vi "PV Main.vi"(10 "Data DVRs":T1, 11 "Config Folder":path) -> ()   [LabVIEW 2018]
uses:
  <vilib>/ORNL/CSEISMIC DDS/CSEISMIC DDS Base/Data Types/Controls/DeviceID.ctl
  Controls/DDS State.ctl
  Controls/Data Type DVRs.ctl
  <vilib>/ORNL/CSEISMIC DDS/CSEISMIC DDS Base/Data Types/IED_Status.ctl
  <vilib>/ORNL/CSEISMIC DDS/CSEISMIC DDS Base/Data Types/Controls/Timestamp.ctl
  <vilib>/ORNL/CSEISMIC DDS/CSEISMIC DDS Base/Data Types/DER_Control.ctl
  <vilib>/ORNL/CSEISMIC DDS/CSEISMIC DDS Base/Data Types/DER_SetPointP.ctl
  <vilib>/ORNL/CSEISMIC DDS/CSEISMIC DDS Base/Data Types/DER_SetPointQ.ctl
  <vilib>/ORNL/CSEISMIC DDS/CSEISMIC DDS Base/Data Types/DER_Measurement.ctl
  <vilib>/ORNL/CSEISMIC DDS/CSEISMIC DDS Base/Data Types/DER_Status.ctl
  <vilib>/ORNL/CSEISMIC DDS/CSEISMIC DDS Base/Data Types/Controls/DroopCurve.ctl
  1ea38d0c-38a7-4a3d-ae1e-65f6e0254380.vi
  8ec4fbad-6e5c-457e-b0e3-a341ac60e8a3.vi
  0ef71f9b-3bca-4440-a5c8-8282c2586051.vi
  9f7c2006-f978-4bec-9c38-bdd34ecae6aa.vi
  3fc4b4bd-7c90-499c-9ed9-e822aa1def77.vi
  ea58e506-6616-4327-a77b-3af52f62fbc1.vi
  89549c33-b0cf-467c-b5c7-b685aa9ebbb0.vi
  4802f4bd-dba4-4fda-a24e-999c1f9497bc.vi
  3edf557d-cbb6-4b9c-94ed-0284affd1f65.vi
  Global Variables/Stop (Global).vi
  Global Variables/DDS States (Global).vi
  Global Variables/Broadcast Topics (Global).vi
  Global Variables/Measurements (Global).vi
  Global Variables/Timeout Topics (Global).vi
  <vilib>/ORNL/CSEISMIC DDS/CSEISMIC DDS Base/CSEISMIC DDS.lvclass
panel:
  out "P_ref":sgl
  out "Q_ref":sgl
  out "P_meas":sgl
  out "Q_meas":sgl
  out "MicrogridID":u8
  out "Error in DDS Loop":bool
  out "DDS Loop error out":errorcluster
  out "PV DDS State":T2=enum."Shutdown"
  out "DDS loop time":u32=105
  out "DeviceID":T3
  out "Enable INV A":bool
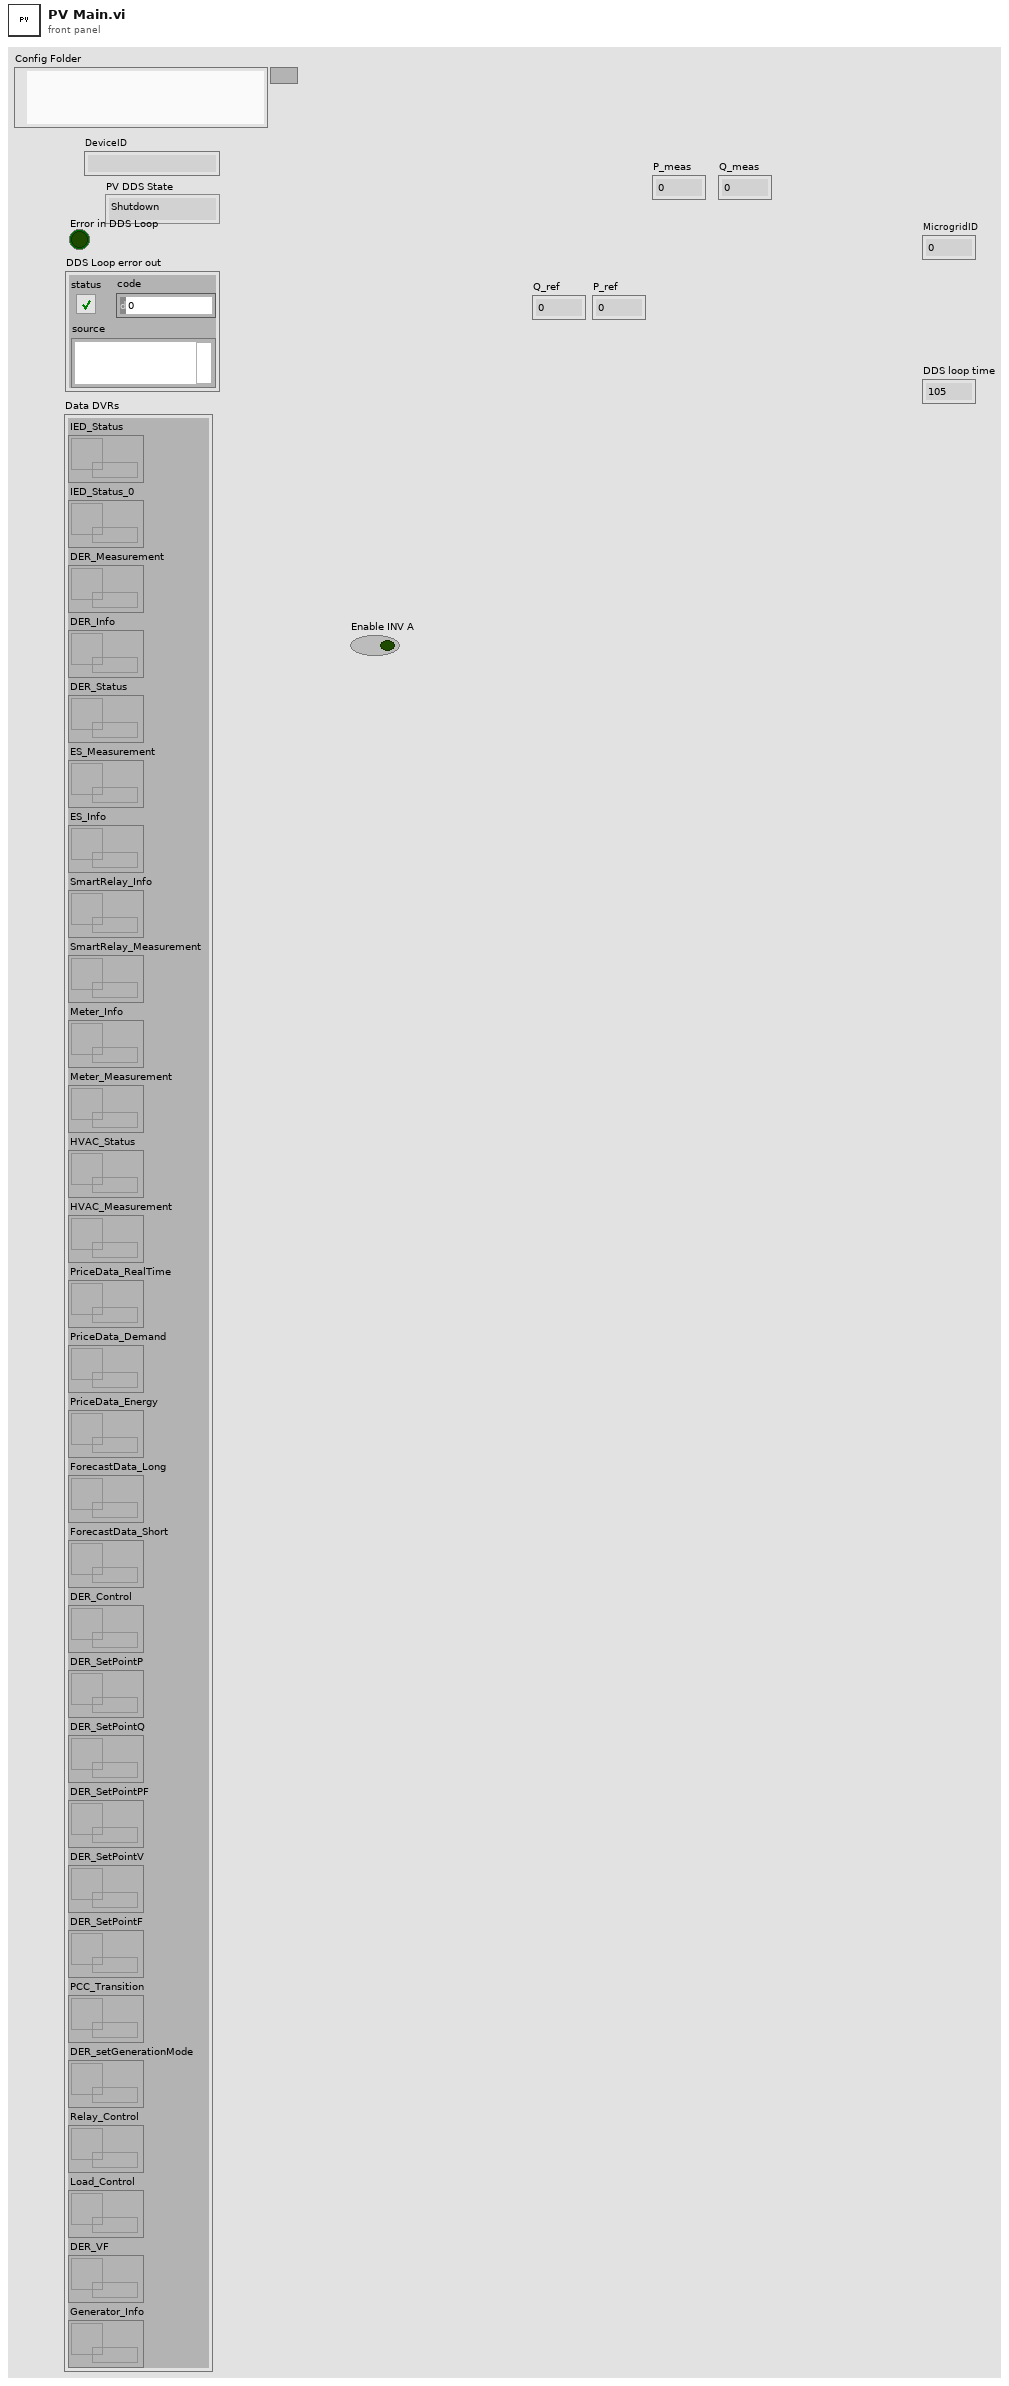
[diagram p1: front panel]
types:
  T1 = typedef "Data Type DVRs.ctl" = cluster{"IED_Status":refnum<data-value>, "IED_Status_0":refnum<data-value>, "DER_Measurement":refnum<data-value>, "DER_Info":refnum<data-value>, "DER_Status":refnum<data-value>, "ES_Measurement":refnum<data-value>, "ES_Info":refnum<data-value>, "SmartRelay_Info":refnum<data-value>, "SmartRelay_Measurement":refnum<data-value>, "Meter_Info":refnum<data-value>, "Meter_Measurement":refnum<data-value>, "HVAC_Status":refnum<data-value>, "HVAC_Measurement":refnum<data-value>, "PriceData_RealTime":refnum<data-value>, "PriceData_Demand":refnum<data-value>, "PriceData_Energy":refnum<data-value>, "ForecastData_Long":refnum<data-value>, "ForecastData_Short":refnum<data-value>, "DER_Control":refnum<data-value>, "DER_SetPointP":refnum<data-value>, "DER_SetPointQ":refnum<data-value>, "DER_SetPointPF":refnum<data-value>, "DER_SetPointV":refnum<data-value>, "DER_SetPointF":refnum<data-value>, "PCC_Transition":refnum<data-value>, "DER_setGenerationMode":refnum<data-value>, "Relay_Control":refnum<data-value>, "Load_Control":refnum<data-value>, "DER_VF":refnum<data-value>, "Generator_Info":refnum<data-value>}
  T2 = typedef "DDS State.ctl" = enum16{"Commissioning", "CheckID", "InitDDS", "ReadDDS", "WriteDDS", "CheckClose", "Close", "Shutdown"}
  T3 = typedef "CSEISMIC DDS.lvlib/CSEISMIC DDS.lvclass/DeviceID.ctl" = string
  T4 = typedef "Scaling Coefficients Cluster.ctl" = cluster{"Measurements":T5, "Setpoints":T6}
  T5 = typedef "Scaling Coefficients Measurements.ctl" = cluster{"Current":dbl, "Voltage":dbl, "Real Power":dbl, "Reactive Power":dbl, "SOC":dbl}
  T6 = typedef "Scaling Coefficients Setpoints.ctl" = cluster{"Voltage":dbl, "Frequency":dbl, "Real Power":dbl, "Reactive Power":dbl}
  T7 = typedef "CSEISMIC DDS.lvlib/CSEISMIC DDS.lvclass/DER_Info.ctl" = cluster{"DeviceID":T3, "LineConfig":u8[], "NominalVoltage(V)":dbl, "PowerRating(kVA)":dbl, "VFControl":bool, "PControl":bool, "QControl":bool, "PFControl":bool, "PVControl":bool, "Droop":bool, "DroopConfigurable":bool, "Unbalanced":bool}
  T8 = typedef "CSEISMIC DDS.lvlib/CSEISMIC DDS.lvclass/Timestamp.ctl" = cluster{"Seconds":u64, "Remainder":u64}
  T9 = typedef "CSEISMIC DDS.lvlib/CSEISMIC DDS.lvclass/IED_Status.ctl" = cluster{"DeviceID":T3, "Timestamp":T8, "MicrogridID":u8, "Active":bool, "Inactive":bool, "Error":i32, "Fault":bool, "ErrorString":string}
  T10 = typedef "CSEISMIC DDS.lvlib/CSEISMIC DDS.lvclass/DER_SetPointQ.ctl" = cluster{"DeviceID":T3, "ReactivePower (kVAR)":dbl[]}
  T11 = typedef "CSEISMIC DDS.lvlib/CSEISMIC DDS.lvclass/DER_SetPointP.ctl" = cluster{"DeviceID":T3, "RealPower (kW)":dbl[]}
  T12 = typedef "CSEISMIC DDS.lvlib/CSEISMIC DDS.lvclass/DER_Control.ctl" = cluster{"DeviceID":T3, "Activate":bool, "Deactivate":bool}
  T13 = typedef "CSEISMIC DDS.lvlib/CSEISMIC DDS.lvclass/DER_Status.ctl" = cluster{"DeviceID":T3, "VFControl":bool, "PControl":bool, "QControl":bool, "PFControl":bool, "PVControl":bool, "Droop":bool, "Unbalanced":bool, "MicrogridVF":bool, "RealDroop(kW)":T14, "ReactiveDroop(kVar)":T14}
  T14 = typedef "CSEISMIC DDS.lvlib/CSEISMIC DDS.lvclass/DroopCurve.ctl" = cluster{"XMin":dbl, "XMax":dbl, "YMin":dbl, "YMax":dbl}
  T15 = typedef "CSEISMIC DDS.lvlib/CSEISMIC DDS.lvclass/DER_Measurement.ctl" = cluster{"DeviceID":T3, "Voltage":dbl[], "Current":dbl[], "RealPower":dbl[], "ReactivePower":dbl[], "LineConfig":u8[], "Frequency":dbl}
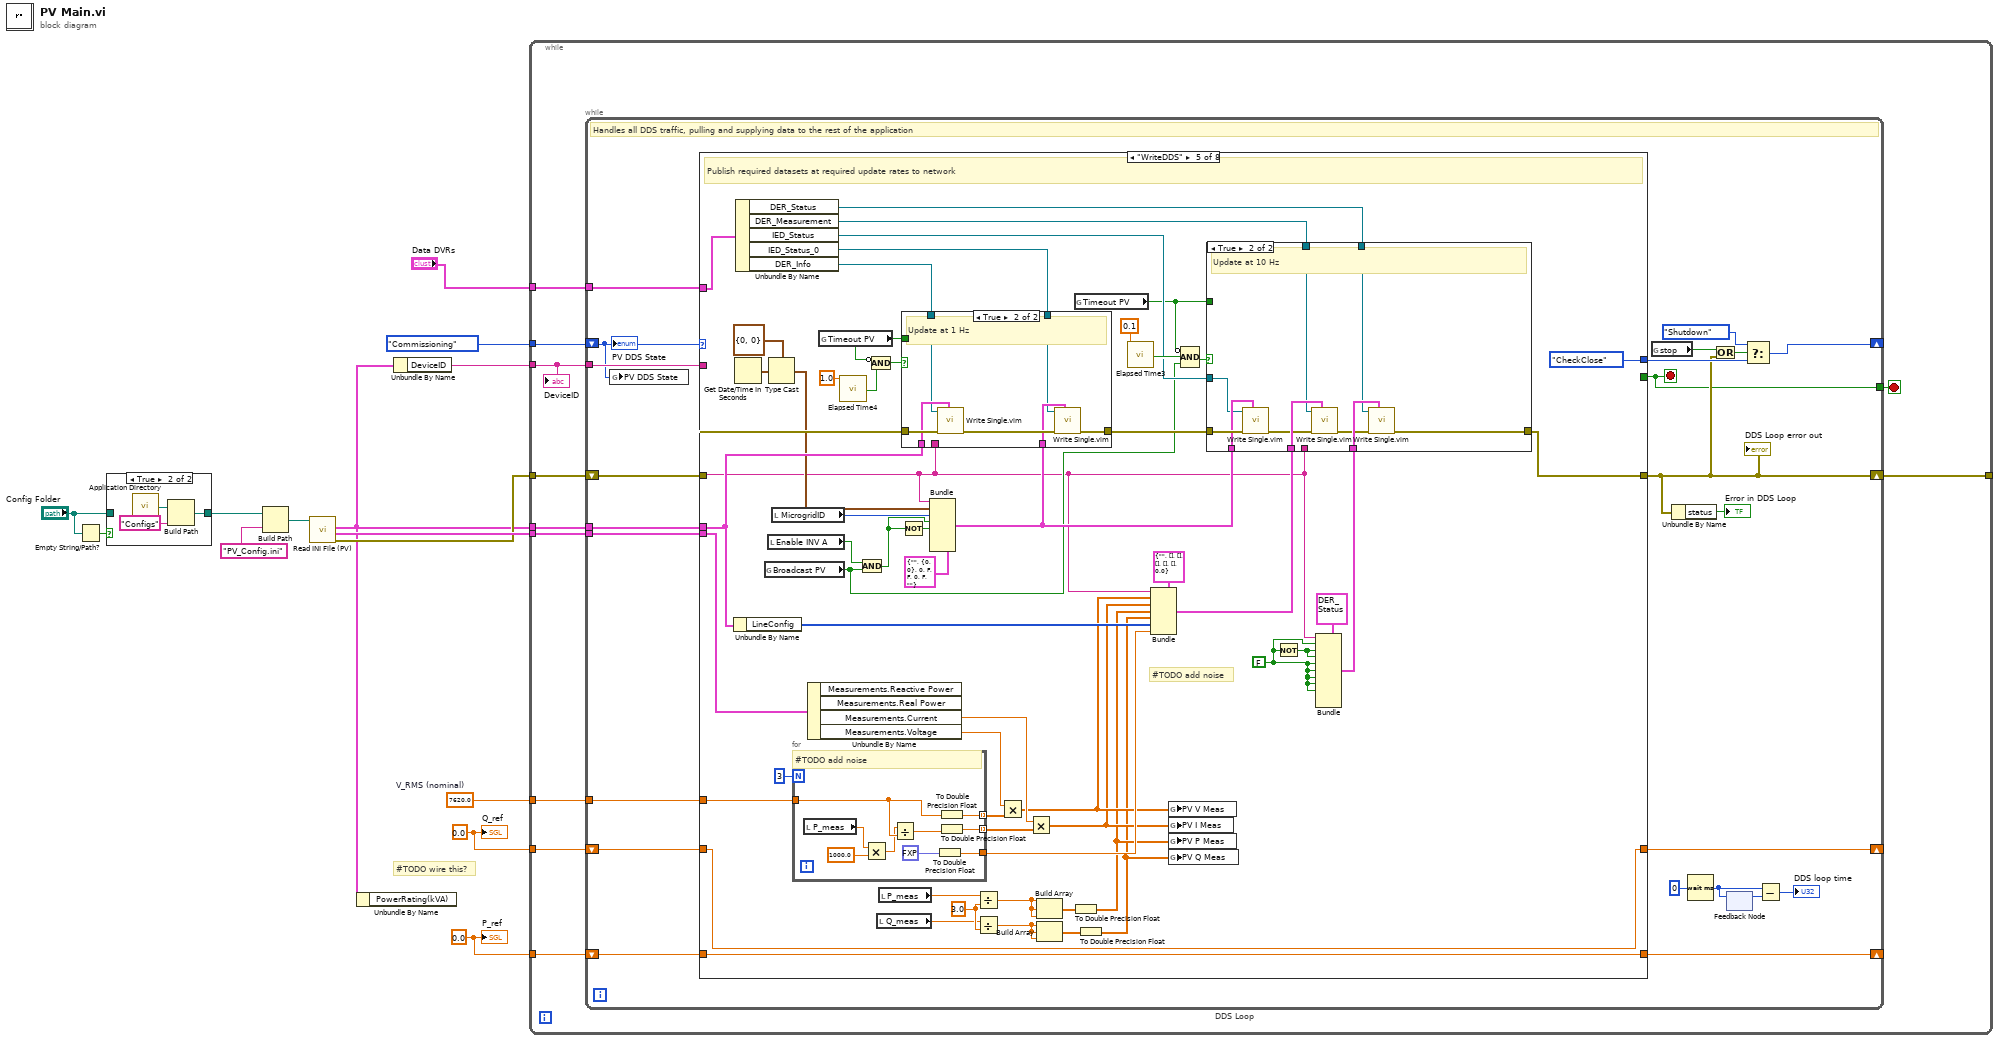
[diagram p0: block diagram]
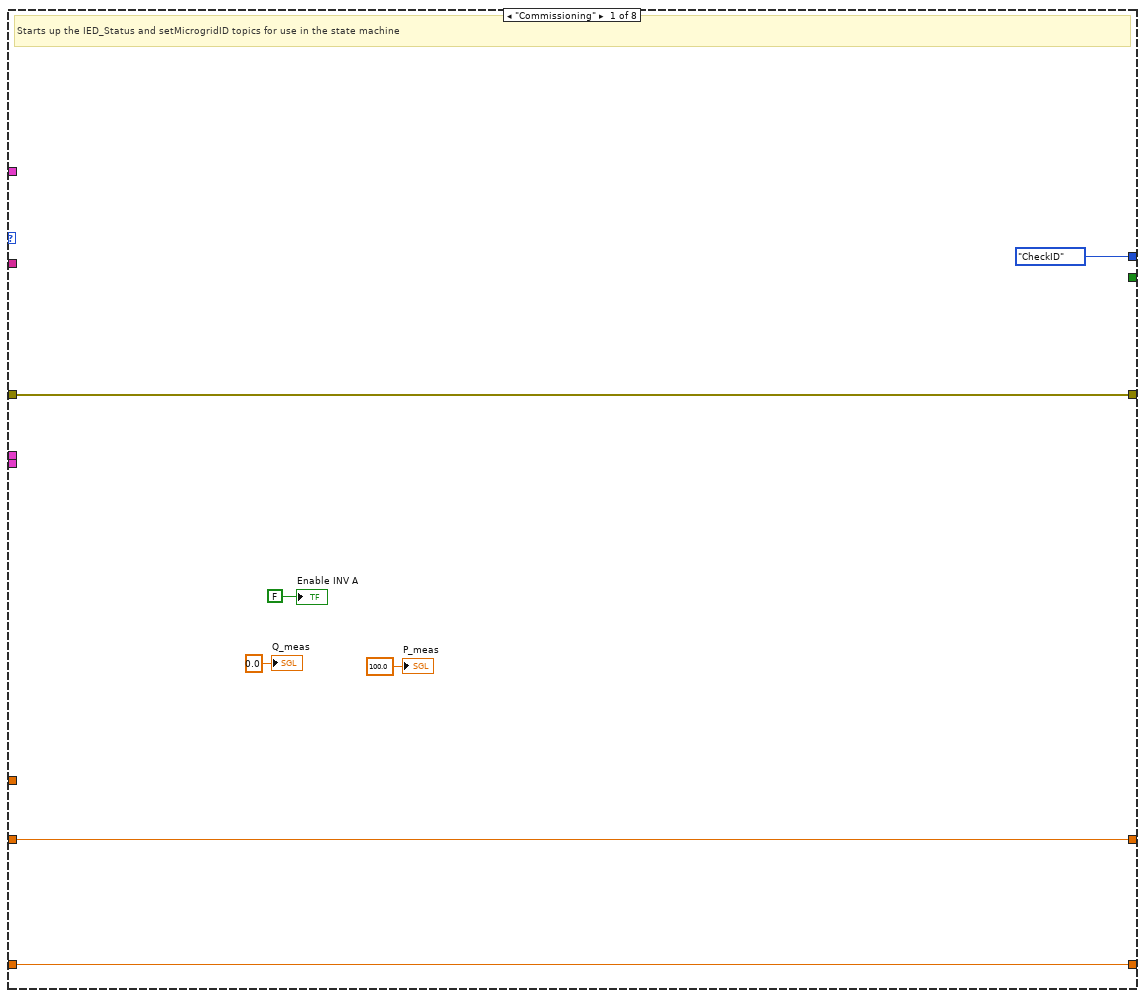
[diagram p2: hidden frame]
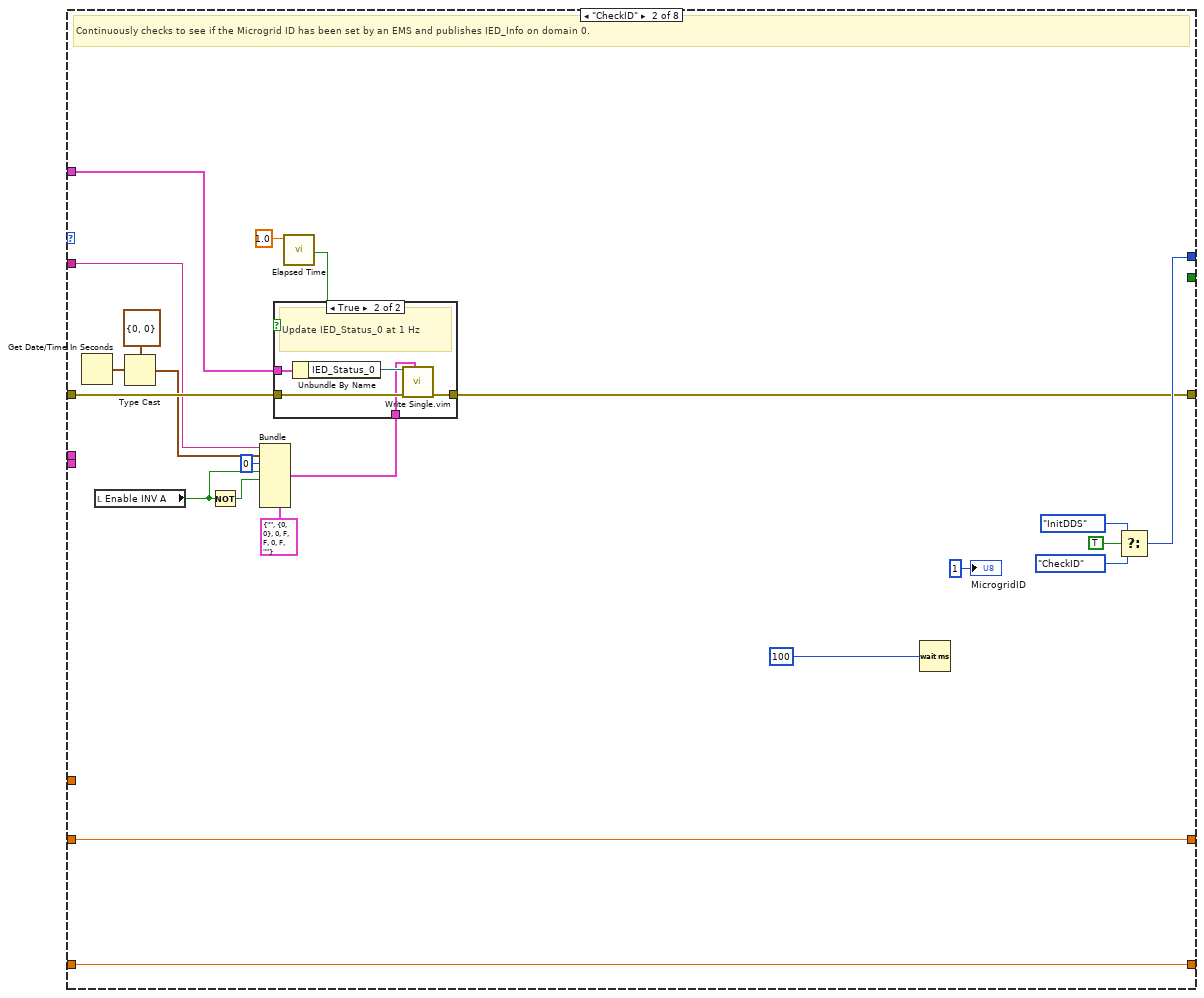
[diagram p3: hidden frame]
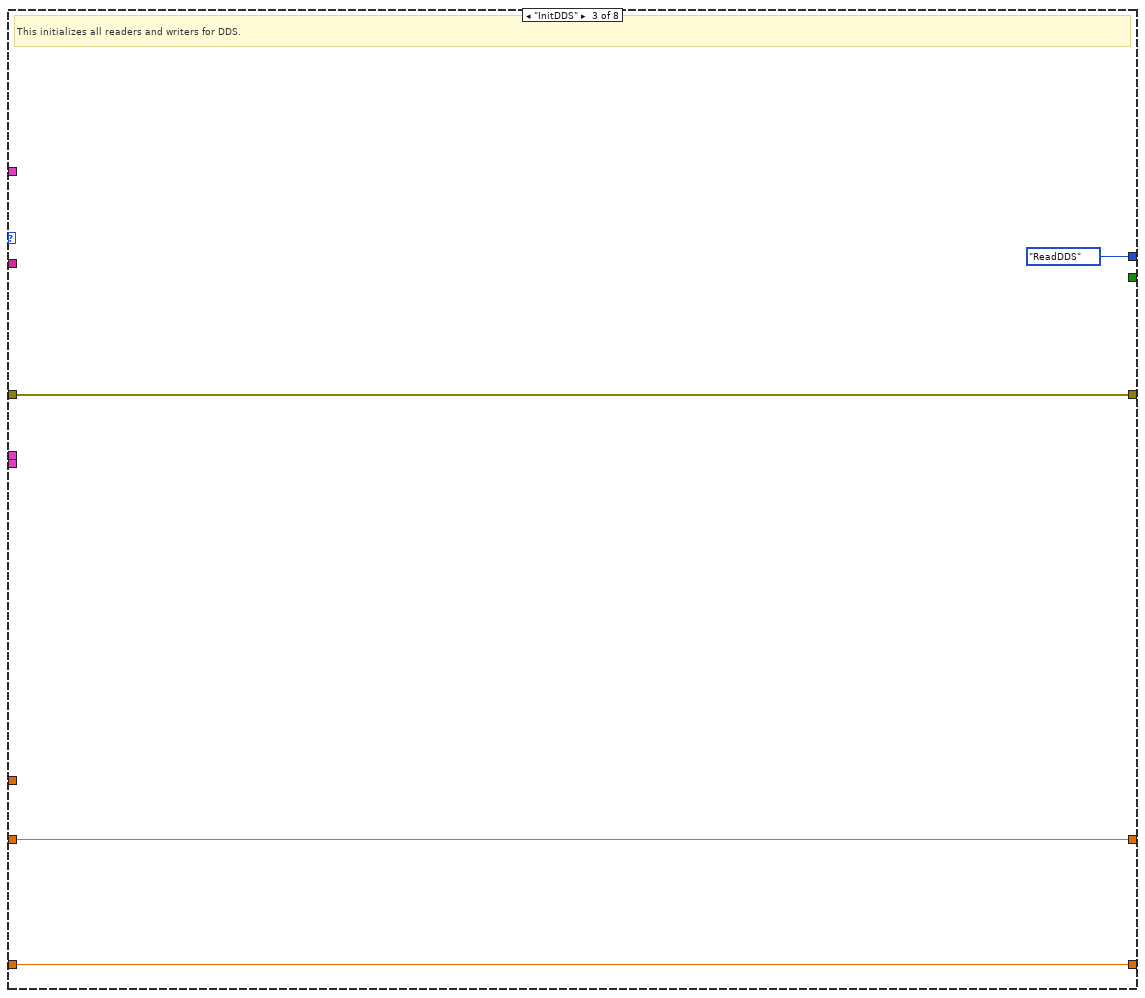
[diagram p5: hidden frame]
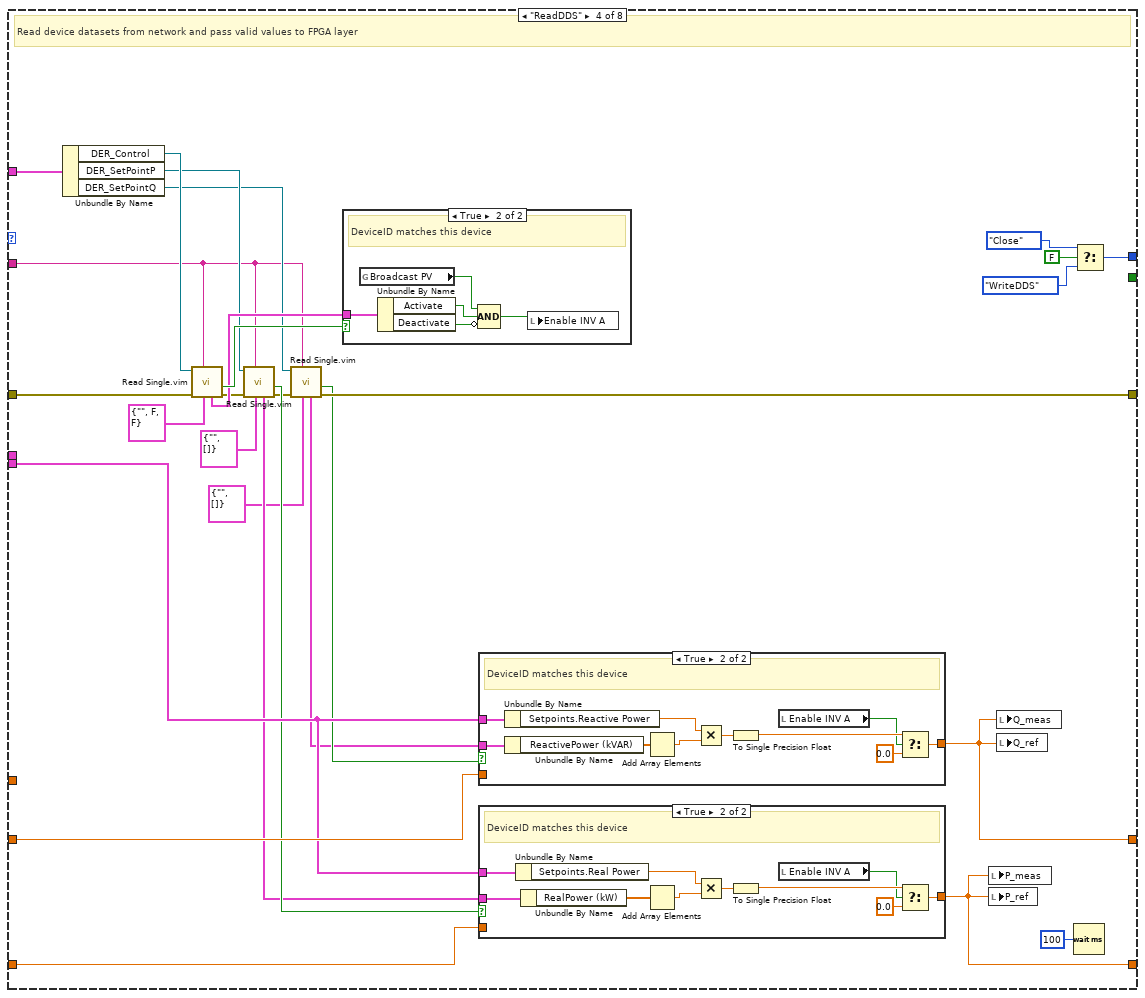
[diagram p6: hidden frame]
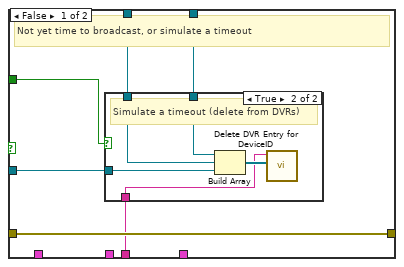
[diagram p10: hidden frame]
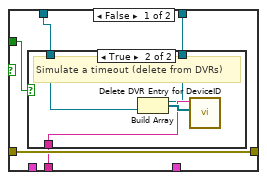
[diagram p12: hidden frame]
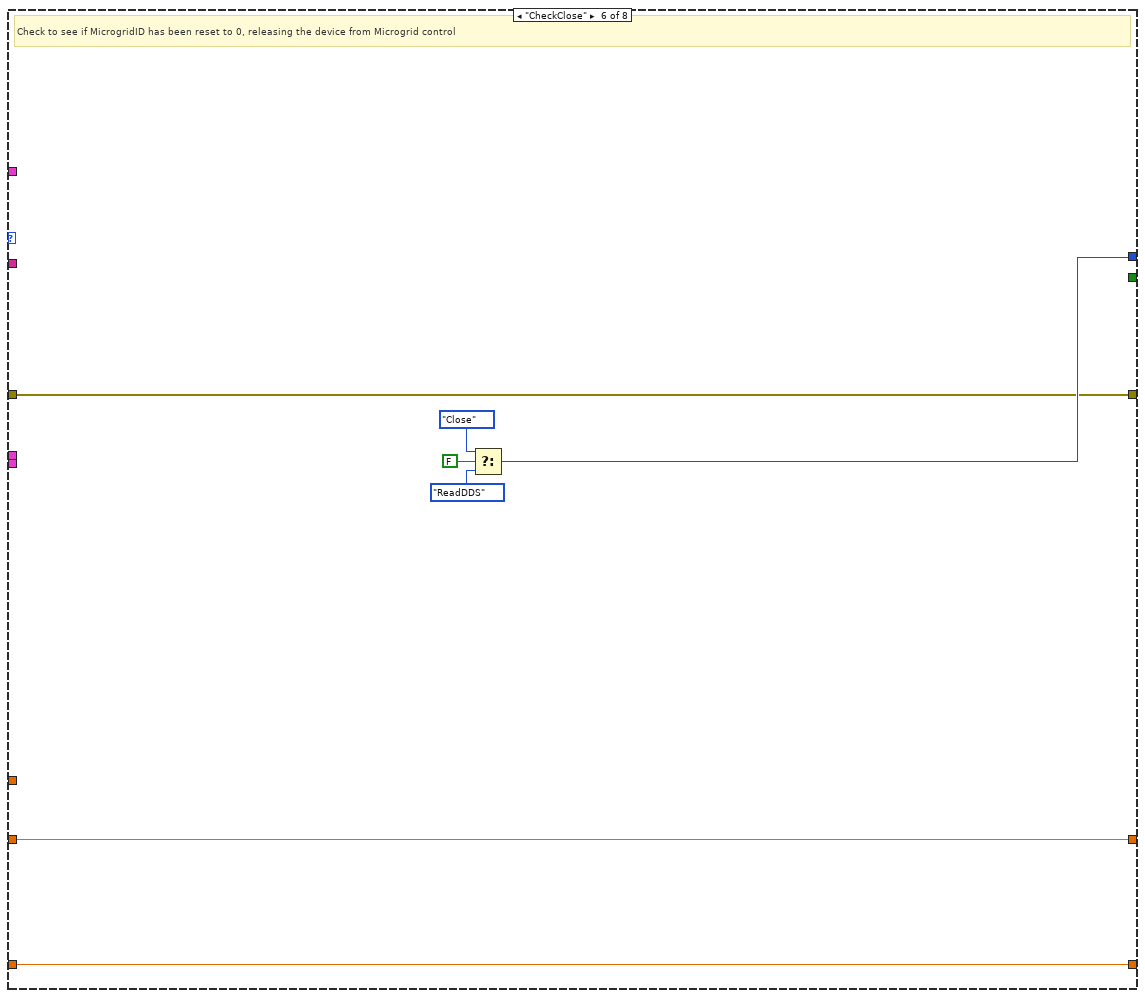
[diagram p14: hidden frame]
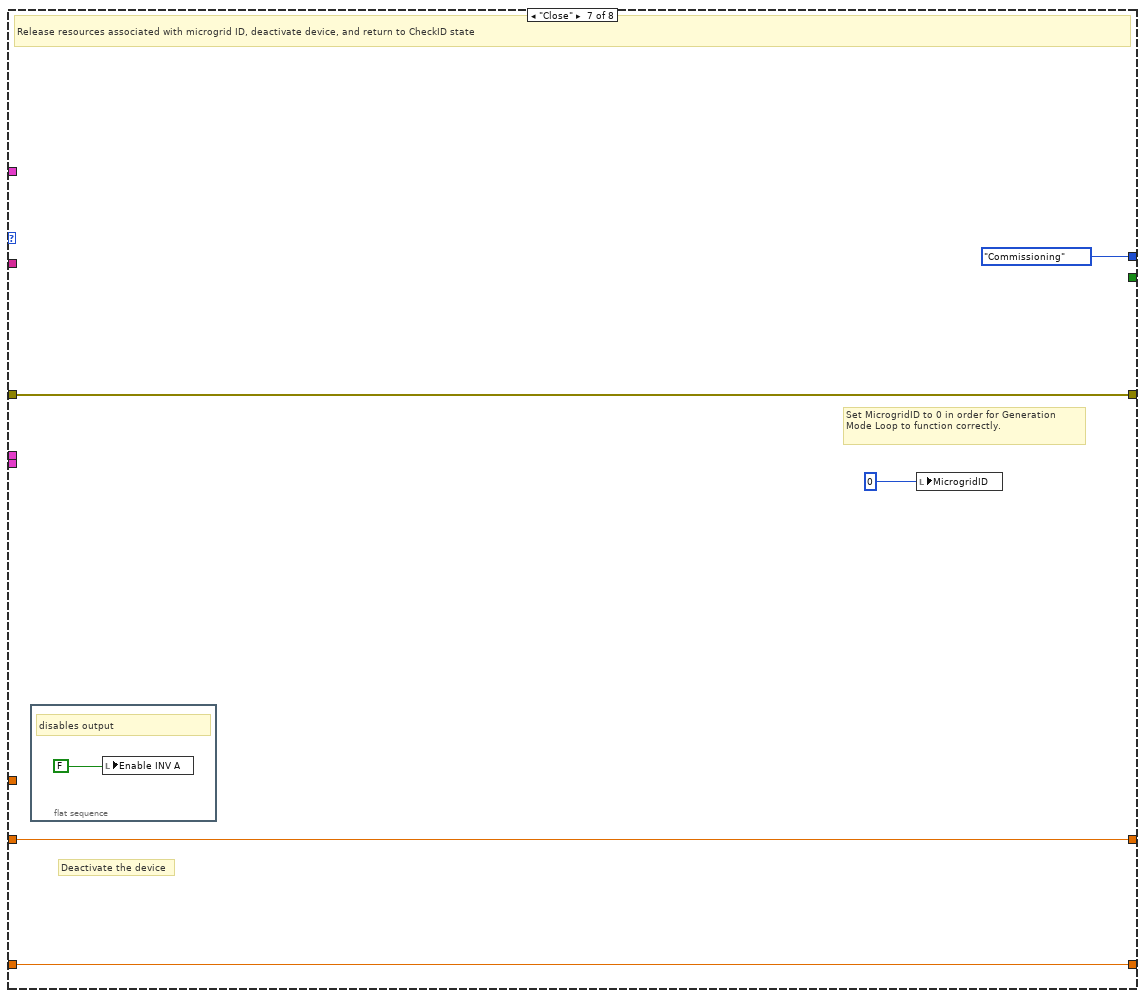
[diagram p15: hidden frame]
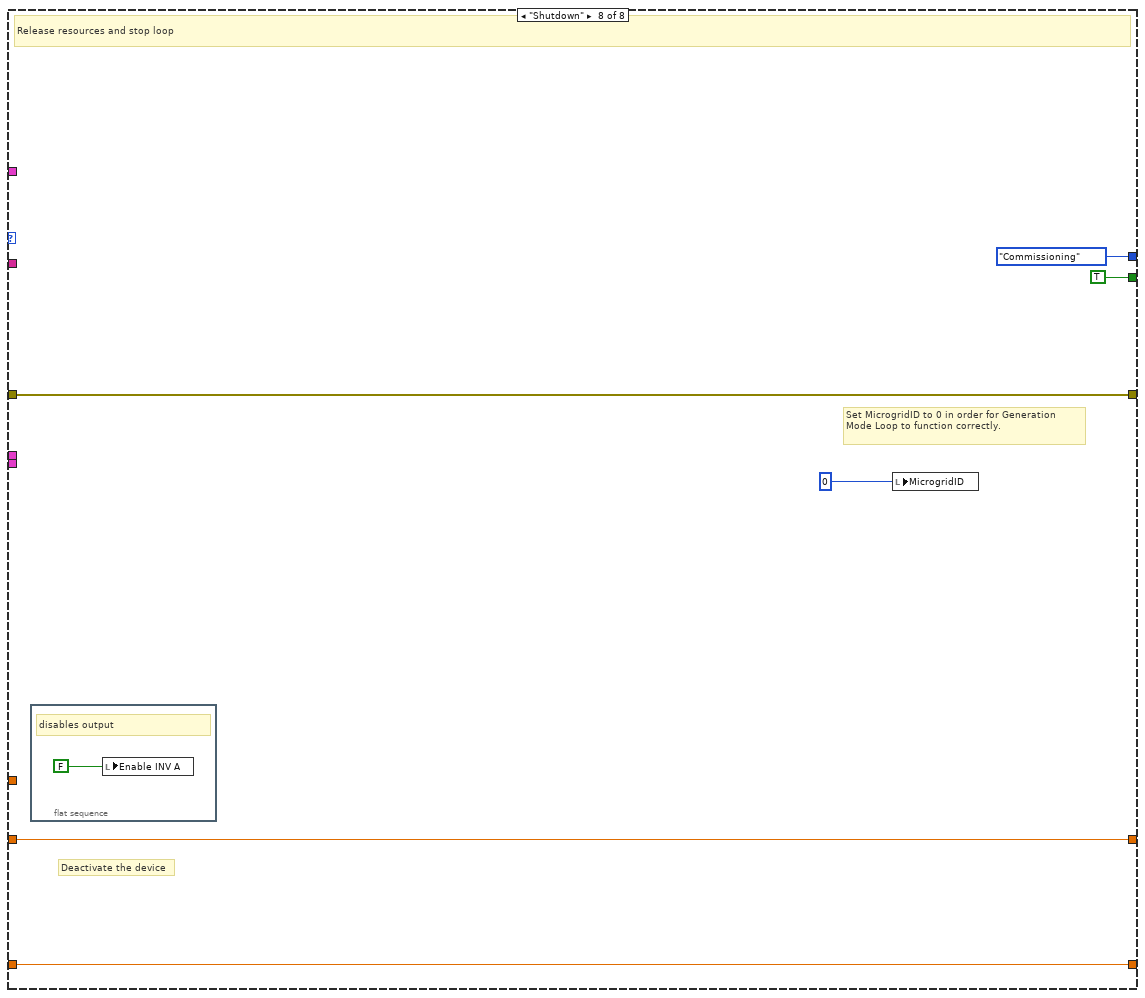
[diagram p16: hidden frame]
diagram:
  w6 = 7620.0  # V_RMS (nominal)
  w7 = sgl 0.0 ("Q_ref")
  w8 = sgl 0.0 ("P_ref")
  # "#TODO wire this?"
  n1 = Empty String/Path?(string/path="Config Folder") -> (empty?=w5:bool)
  n2 = case shown="True" w5 {
    tunnel: [w15 w16] -> w4
    tunnel: "Config Folder" -> [w15 _]
    frame False {
    }
    frame True {
      n3 = call <vilib>:"Application Directory.vi"() -> ("Application Directory"=w18:path)
      n4 = Build Path(base path=w18, name or relative path="Configs") -> (appended path=w16:path)
    }
  }
  n5 = Build Path(base path=w4, name or relative path="PV_Config.ini") -> (appended path=w13:path)
  n6 = call "Read INI File (PV).vi"("Path"=w13) -> ("error out"=w10:errorcluster, "Scaling Coefficients"=w11:T4, "DER_Info"=w1:T7)  [unwired: 8 in]
  n7 = Unbundle By Name(w1) -> ()  [unwired: 1 out]
  n8 = Unbundle By Name(w1) -> ("DeviceID"=w12:T3)
  n9 = while {
    tunnel: DDS_State."Commissioning" ("DDS State 2") -> [w29]
    tunnel: w1 -> [w28]
    tunnel: w10 -> [w27]
    tunnel: w11 -> [w26]
    tunnel: w12 -> [w25]
    tunnel: [w23] -> _
    tunnel: w8 -> [w22]
    tunnel: w7 -> [w21]
    tunnel: w6 -> [w20]
    tunnel: "Data DVRs" -> [w19]
    stop <- w24 stop-if-true
    n10 = while "DDS Loop" {
      shift-right: [w49] -> _
      shift-left: w29 -> [w30]
      tunnel: w25 -> [w52]
      shift-right: [w44] -> w23
      shift-left: w27 -> [w51]
      tunnel: w28 -> [w50]
      tunnel: w26 -> [w45]
      tunnel: [w42] -> w24
      shift-right: [w36] -> _
      shift-left: w22 -> [w35]
      shift-right: [w34] -> _
      shift-left: w21 -> [w33]
      tunnel: w20 -> [w32]
      tunnel: w19 -> [w37]
      stop <- w42 stop-if-true
      # "Handles all DDS traffic, pulling and supplying data to the rest of the application"
      n11 = global write "DDS States (Global).vi" "PV DDS State"(w30) -> ()
      n12 = case shown="\"WriteDDS\"" w30 {
        tunnel: [DDS_State."CheckID" w76 DDS_State."ReadDDS" w117 DDS_State."CheckClose" w255 DDS_State."Commissioning" ("f") DDS_State."Commissioning" ("f")] -> w48
        tunnel: [w58 w67 w90 w96 w198 w254 w261 w268] -> w44
        tunnel: w52 -> [_ w66 _ w94 w147 _ _ _]
        tunnel: w51 -> [w58 w79 w90 w108 w203 w254 w261 w268]
        tunnel: w50 -> [_ _ _ _ w195 _ _ _]
        tunnel: [_ _ _ _ _ _ _ TRUE] -> w42
        tunnel: w45 -> [_ _ _ w113 w192 _ _ _]
        tunnel: w37 -> [_ w62 _ w109 w161 _ _ _]
        tunnel: [w57 w65 w89 w111 w176 w253 w259 w265] -> w36
        tunnel: w35 -> [w57 w65 w89 w112 w176 w253 w259 w265]
        tunnel: [w56 w64 w88 w114 w175 w252 w258 w264] -> w34
        tunnel: w33 -> [w56 w64 w88 w115 w175 w252 w258 w264]
        tunnel: w32 -> [_ _ _ _ w170 _ _ _]
        frame "Commissioning" {
          # "Starts up the IED_Status and setMicrogridID topics for use in the state machine"
          "Q_meas" <- sgl 0.0 ("Q_meas")
          "P_meas" <- sgl 100.0 ("P_meas")
          "Enable INV A" <- FALSE ("Enable INV A")
        }
        frame "CheckID" {
          # "Continuously checks to see if the Microgrid ID has been set by an EMS and publishes IED_Info on domain 0."
          n13 = Get Date/Time In Seconds() -> (seconds since 1Jan1904=w72:timestamp)
          n14 = local read "Enable INV A"() -> (w63:bool)
          n15 = Type Cast(type=T8 {"Seconds"=0, "Remainder"=0} ("Timestamp"), x=w72) -> (*(type *) &x=w70:T8)
          n16 = Not(x=w63) -> (.not. x?=w68:bool)
          n17 = Bundle(cluster=T9 {"DeviceID"="", "Timestamp"={"Seconds"=0, "Remainder"=0}, "MicrogridID"=0, "Active"=FALSE, "Inactive"=FALSE, "Error"=0, "Fault"=FALSE, "ErrorString"=""} ("output cluster"), "DeviceID"=w66, "Timestamp"=w70, "MicrogridID"=u8 0, "Active"=w63, "Inactive"=w68) -> (w80:T9)  [unwired: 3 in]
          n18 = call "Elapsed Time"("Time Target (s)"=1.0) -> ("Time has Elapsed"=w75:bool)  [unwired: 11 in, 7 out]
          n19 = case shown="True" w75 {
            tunnel: w80 -> [_ w83]
            tunnel: [w82 w86] -> w67
            tunnel: w79 -> [w82 w87]
            tunnel: w62 -> [_ w85]
            frame False {
            }
            frame True {
              # "Update IED_Status_0 at 1 Hz"
              n20 = Unbundle By Name(w85) -> ("IED_Status_0"=w84:refnum<data-value>)
              n21 = call "Write Single.vim"("Data Element"=w83, "error in"=w87, "Data DVR"=w84) -> ("dup error out"=w86:errorcluster)  [unwired: 8 in]
            }
          }
          n22 = Wait (ms)(milliseconds to wait=u32 100) -> ()  [unwired: 1 out]
          n23 = Select(t=DDS_State."InitDDS", s=TRUE, f=DDS_State."CheckID") -> (s? t:f=w76:T2)
          "MicrogridID" <- u8 1 ("MicrogridID")
        }
        frame "InitDDS" {
          # "This initializes all readers and writers for DDS."
        }
        frame "ReadDDS" {
          # "Read device datasets from network and pass valid values to FPGA layer"
          n24 = Unbundle By Name(w109) -> ("DER_Control"=w106:refnum<data-value>, "DER_SetPointP"=w100:refnum<data-value>, "DER_SetPointQ"=w98:refnum<data-value>)
          n25 = call "Read Single.vim"("Data Type"=T12 {"DeviceID"="", "Activate"=FALSE, "Deactivate"=FALSE} ("DER_Control"), "DeviceID"=w94, "error in"=w108, "Data DVR"=w106) -> ("dup error out"=w103:errorcluster, "Valid"=w105:bool, "Data Element"=w104:T12)  [unwired: 5 in]
          n26 = call "Read Single.vim"("Data Type"=T11 {"DeviceID"="", "RealPower (kW)"=[]} ("DER_SetPointP"), "DeviceID"=w94, "error in"=w103, "Data DVR"=w100) -> ("dup error out"=w97:errorcluster, "Valid"=w102:bool, "Data Element"=w99:T11)  [unwired: 5 in]
          n27 = call "Read Single.vim"("Data Type"=T10 {"DeviceID"="", "ReactivePower (kVAR)"=[]} ("DER_SetPointQ"), "DeviceID"=w94, "error in"=w97, "Data DVR"=w98) -> ("dup error out"=w96:errorcluster, "Valid"=w93:bool, "Data Element"=w92:T10)  [unwired: 5 in]
          n28 = case shown="True" w105 {
            tunnel: w104 -> [_ w146]
            frame False {
              # "Non-matching DeviceID"
            }
            frame True {
              # "DeviceID matches this device"
              n29 = global read "Broadcast Topics (Global).vi" "Broadcast PV"() -> (w142:bool)
              n30 = Unbundle By Name(w146) -> ("Activate"=w144:bool, "Deactivate"=w145:bool)
              n31 = Compound Arithmetic op=AND(w142, w144, invert w145) -> (w143:bool)
              n32 = local write "Enable INV A"(w143) -> ()
            }
          }
          n33 = case shown="True" w93 {
            tunnel: w92 -> [_ w141]
            tunnel: w113 -> [_ w140]
            tunnel: [w131 w133] -> w114
            tunnel: w115 -> [w131 _]
            frame False {
              # "Non-matching DeviceID"
            }
            frame True {
              # "DeviceID matches this device"
              n34 = Unbundle By Name(w140) -> ("Setpoints.Reactive Power"=w137:dbl)
              n35 = Unbundle By Name(w141) -> ("ReactivePower (kVAR)"=w139:dbl[])
              n36 = Add Array Elements(numeric array=w139) -> (sum=w138:dbl)
              n37 = Multiply(x=w137, y=w138) -> (x*y=w136:dbl)
              n38 = To Single Precision Float(number=w136) -> (single precision float=w135:sgl)
              n39 = local read "Enable INV A"() -> (w132:bool)
              n40 = Select(t=w135, s=w132, f=sgl 0.0) -> (s? t:f=w133:sgl)
            }
          }
          n41 = case shown="True" w102 {
            tunnel: w99 -> [_ w130]
            tunnel: w113 -> [_ w129]
            tunnel: [w120 w122] -> w111
            tunnel: w112 -> [w120 _]
            frame False {
              # "Non-matching DeviceID"
            }
            frame True {
              # "DeviceID matches this device"
              n42 = Unbundle By Name(w129) -> ("Setpoints.Real Power"=w126:dbl)
              n43 = Unbundle By Name(w130) -> ("RealPower (kW)"=w128:dbl[])
              n44 = Add Array Elements(numeric array=w128) -> (sum=w127:dbl)
              n45 = Multiply(x=w126, y=w127) -> (x*y=w125:dbl)
              n46 = To Single Precision Float(number=w125) -> (single precision float=w124:sgl)
              n47 = local read "Enable INV A"() -> (w121:bool)
              n48 = Select(t=w124, s=w121, f=sgl 0.0) -> (s? t:f=w122:sgl)
            }
          }
          n49 = local write "P_meas"(w111) -> ()
          n50 = local write "P_ref"(w111) -> ()
          n51 = local write "Q_meas"(w114) -> ()
          n52 = local write "Q_ref"(w114) -> ()
          n53 = Wait (ms)(milliseconds to wait=u32 100) -> ()  [unwired: 1 out]
          n54 = Select(t=DDS_State."Close", s=FALSE, f=DDS_State."WriteDDS") -> (s? t:f=w117:T2)
        }
        frame "WriteDDS" {
          w179 = sgl 3.0 ("y")
          w168 = FALSE ("PFControl")
          # "#TODO add noise"
          # "Publish required datasets at required update rates to network"
          n55 = Unbundle By Name(w195) -> ("LineConfig"=w194:u8[])
          n56 = Get Date/Time In Seconds() -> (seconds since 1Jan1904=w187:timestamp)
          n57 = Unbundle By Name(w161) -> ("DER_Status"=w156:refnum<data-value>, "DER_Measurement"=w157:refnum<data-value>, "IED_Status"=w158:refnum<data-value>, "IED_Status_0"=w159:refnum<data-value>, "DER_Info"=w160:refnum<data-value>)
          n58 = global read "Broadcast Topics (Global).vi" "Broadcast PV"() -> (w153:bool)
          n59 = local read "Enable INV A"() -> (w155:bool)
          n60 = Type Cast(type=T8 {"Seconds"=0, "Remainder"=0} ("Timestamp"), x=w187) -> (*(type *) &x=w184:T8)
          n61 = local read "MicrogridID"() -> (w183:u8)
          n62 = for {
            N: 3 -> [_]
            tunnel: [w213] -> w191 mode=indexing
            tunnel: [w212] -> w190 mode=indexing
            tunnel: w170 -> [w210]
            tunnel: [w209] -> w169
            # "#TODO add noise"
            n63 = local read "P_meas"() -> (w207:sgl)
            n64 = Multiply(x=w207, y=sgl 1000.0) -> (x*y=w206:sgl)
            n65 = Divide(x=w206, y=w210) -> (x/y=w211:dbl)
            n66 = To Double Precision Float(number=fxp<+,20,6> 60.0 ("f_islanded")) -> (double precision float=w209:dbl)
            n67 = To Double Precision Float(number=w210) -> (double precision float=w213:dbl)
            n68 = To Double Precision Float(number=w211) -> (double precision float=w212:dbl)
          }
          n69 = Unbundle By Name(w192) -> ("Measurements.Current"=w188:dbl, "Measurements.Voltage"=w189:dbl)  [unwired: 2 out]
          n70 = global read "Timeout Topics (Global).vi" "Timeout PV"() -> (w148:bool)
          n71 = call "Elapsed Time4"("Time Target (s)"=1.0) -> ("Time has Elapsed"=w150:bool)  [unwired: 11 in, 7 out]
          n72 = And(x=w155, y=w153) -> (x .and. y?=w154:bool)
          n73 = Compound Arithmetic op=AND(invert w148, w150) -> (w149:bool)
          n74 = local read "Q_meas"() -> (w173:sgl)
          n75 = local read "P_meas"() -> (w174:sgl)
          n76 = Not(x=w154) -> (.not. x?=w182:bool)
          n77 = Bundle(cluster=T9 {"DeviceID"="", "Timestamp"={"Seconds"=0, "Remainder"=0}, "MicrogridID"=0, "Active"=FALSE, "Inactive"=FALSE, "Error"=0, "Fault"=FALSE, "ErrorString"=""} ("IED_Status"), "DeviceID"=w147, "Timestamp"=w184, "MicrogridID"=w183, "Active"=w154, "Inactive"=w182) -> (w201:T9)  [unwired: 3 in]
          n78 = case shown="True" w149 {
            tunnel: w203 -> [w239 w250]
            tunnel: [w239 w244] -> w202
            tunnel: w201 -> [_ w246]
            tunnel: w195 -> [_ w249]
            tunnel: w160 -> [w237 w248]
            tunnel: w159 -> [w236 w245]
            tunnel: w148 -> [w238 _]
            tunnel: w147 -> [w235 _]
            frame False {
              n79 = case shown="True" w238 {
                tunnel: w237 -> [_ w242]
                tunnel: w235 -> [_ w241]
                tunnel: w236 -> [_ w240]
                frame False {
                  # "Not time to broadcast yet"
                }
                frame True {
                  # "Simulate a timeout (delete from DVRs)"
                  n80 = Build Array(w240, w242) -> (w243:refnum<data-value>[])
                  n81 = call "Delete DVR Entry for DeviceID.vi"("DVR Array"=w243, "DeviceID"=w241) -> ()  [unwired: 10 in]
                }
              }
            }
            frame True {
              # "Update at 1 Hz"
              n82 = call "Write Single.vim"("Data Element"=w249, "error in"=w250, "Data DVR"=w248) -> ("dup error out"=w247:errorcluster)  [unwired: 8 in]
              n83 = call "Write Single.vim"("Data Element"=w246, "error in"=w247, "Data DVR"=w245) -> ("dup error out"=w244:errorcluster)  [unwired: 8 in]
            }
          }
          n84 = Divide(x=w174, y=w179) -> (x/y=w178:sgl)
          n85 = Divide(x=w173, y=w179) -> (x/y=w177:sgl)
          n86 = Multiply(x=w189, y=w191) -> (x*y=w167:dbl[])
          n87 = Multiply(x=w188, y=w190) -> (x*y=w166:dbl[])
          n88 = Build Array(w178, w178, w178) -> (w165:sgl[])
          n89 = Build Array(w177, w177, w177) -> (w164:sgl[])
          n90 = To Double Precision Float(number=w165) -> (double precision float=w163:dbl[])
          n91 = global read "Timeout Topics (Global).vi" "Timeout PV"() -> (w151:bool)
          n92 = To Double Precision Float(number=w164) -> (double precision float=w162:dbl[])
          n93 = call "Elapsed Time3"("Time Target (s)"=0.1) -> ("Time has Elapsed"=w196:bool)  [unwired: 11 in, 7 out]
          n94 = Bundle(cluster=T15 {"DeviceID"="", "Voltage"=[], "Current"=[], "RealPower"=[], "ReactivePower"=[], "LineConfig"=[], "Frequency"=0.0} ("DER_Measurement"), "DeviceID"=w147, "Voltage"=w167, "Current"=w166, "RealPower"=w163, "ReactivePower"=w162, "LineConfig"=w194, "Frequency"=w169) -> (w200:T15)
          n95 = global write "Measurements (Global).vi" "PV V Meas"(w167) -> ()
          n96 = global write "Measurements (Global).vi" "PV I Meas"(w166) -> ()
          n97 = global write "Measurements (Global).vi" "PV P Meas"(w163) -> ()
          n98 = global write "Measurements (Global).vi" "PV Q Meas"(w162) -> ()
          n99 = Compound Arithmetic op=AND(invert w151, w196, w153) -> (w152:bool)
          n100 = Not(x=w168) -> (.not. x?=w172:bool)
          n101 = Bundle(cluster=T13 {"DeviceID"="", "VFControl"=FALSE, "PControl"=FALSE, "QControl"=FALSE, "PFControl"=FALSE, "PVControl"=FALSE, "Droop"=FALSE, "Unbalanced"=FALSE, "MicrogridVF"=FALSE, "RealDroop(kW)"={"XMin"=0.0, "XMax"=0.0, "YMin"=0.0, "YMax"=0.0}, "ReactiveDroop(kVar)"={"XMin"=0.0, "XMax"=0.0, "YMin"=0.0, "YMax"=0.0}} ("DER_Status"), "DeviceID"=w147, "VFControl"=w168, "PControl"=w172, "QControl"=w172, "PFControl"=w168, "PVControl"=w168, "Droop"=w168, "Unbalanced"=w168, "MicrogridVF"=w168) -> (w199:T13)  [unwired: 2 in]
          n102 = case shown="True" w152 {
            tunnel: w202 -> [w219 w234]
            tunnel: w201 -> [_ w233]
            tunnel: w200 -> [_ w231]
            tunnel: w199 -> [_ w228]
            tunnel: [w219 w226] -> w198
            tunnel: w158 -> [w218 w232]
            tunnel: w157 -> [w217 w230]
            tunnel: w156 -> [w215 w227]
            tunnel: w147 -> [w216 _]
            tunnel: w151 -> [w214 _]
            frame False {
              # "Not yet time to broadcast, or simulate a timeout"
              n103 = case shown="True" w214 {
                tunnel: w218 -> [_ w221]
                tunnel: w217 -> [_ w222]
                tunnel: w216 -> [_ w220]
                tunnel: w215 -> [_ w223]
                frame False {
                  # "Not time to broadcast yet"
                }
                frame True {
                  # "Simulate a timeout (delete from DVRs)"
                  n104 = Build Array(w223, w222, w221) -> (w224:refnum<data-value>[])
                  n105 = call "Delete DVR Entry for DeviceID.vi"("DVR Array"=w224, "DeviceID"=w220) -> ()  [unwired: 10 in]
                }
              }
            }
            frame True {
              # "Update at 10 Hz"
              n106 = call "Write Single.vim"("Data Element"=w233, "error in"=w234, "Data DVR"=w232) -> ("dup error out"=w229:errorcluster)  [unwired: 8 in]
              n107 = call "Write Single.vim"("Data Element"=w231, "error in"=w229, "Data DVR"=w230) -> ("dup error out"=w225:errorcluster)  [unwired: 8 in]
              n108 = call "Write Single.vim"("Data Element"=w228, "error in"=w225, "Data DVR"=w227) -> ("dup error out"=w226:errorcluster)  [unwired: 8 in]
            }
          }
        }
        frame "CheckClose" {
          # "Check to see if MicrogridID has been reset to 0, releasing the device from Microgrid control"
          n109 = Select(t=DDS_State."Close", s=FALSE, f=DDS_State."ReadDDS") -> (s? t:f=w255:T2)
        }
        frame "Close" {
          # "Set MicrogridID to 0 in order for Generation Mode Loop to function correctly."
          # "Deactivate the device"
          # "Release resources associated with microgrid ID, deactivate device, and return to CheckID state"
          n110 = flat-sequence {
            frame #0 {
              # "disables output"
              n111 = local write "Enable INV A"(FALSE ("PWM Enabled")) -> ()
            }
          }
          n112 = local write "MicrogridID"(u8 0 ("MicrogridID")) -> ()
        }
        frame "Shutdown" {
          # "Set MicrogridID to 0 in order for Generation Mode Loop to function correctly."
          # "Deactivate the device"
          # "Release resources and stop loop"
          n113 = flat-sequence {
            frame #0 {
              # "disables output"
              n114 = local write "Enable INV A"(FALSE ("PWM Enabled")) -> ()
            }
          }
          n115 = local write "MicrogridID"(u8 0 ("MicrogridID")) -> ()
        }
      }
      "DDS Loop error out" <- w44
      n116 = global read "Stop (Global).vi" "stop"() -> (w31:bool)
      n117 = Unbundle By Name(w44) -> ("status"=→"Error in DDS Loop":bool)
      n118 = Wait (ms)(milliseconds to wait=u32 0) -> (millisecond timer value=w40:u32)
      n119 = Or(x=w31, y=w44) -> (x .or. y?=w46:bool)
      n120 = feedback #1() -> (w39:u32)  [unwired: 1 in]
      n121 = feedback-in #1(w40) -> ()
      n122 = Select(t=DDS_State."Shutdown", s=w46, f=w48) -> (s? t:f=w49:T2)
      n123 = Subtract(x=w40, y=w39) -> (x-y=→"DDS loop time":u32)
      "PV DDS State" <- w30
    }
    "DeviceID" <- w25
  }
  "Q_ref" <- w7
  "P_ref" <- w8
